vi "Ultrasonic.vi"(0 "COM":refnum<visa-resource-name>, 1 "Timeout (ms)":u32=500, 5 "Function":T2(ring)=enum."SendWaitRead", 7 "Send":string(combo), 9 "Baudrate":u32=115200, 11 "error in (no error)":errorcluster, 12 "Read regular":string="\n") -> (4 "ReceiveString":string, 6 "welding results  cluster":T1, 15 "error out":errorcluster)   [LabVIEW 2020, in "ultrasonic welding machine.lvlib"]
uses:
  ultrasonic welding machine.lvlib
  <vilib>/Instr/_visa.llb/VISA Set IO Buffer Mask.ctl
  <vilib>/Instr/_visa.llb/VISA Flush IO Buffer Mask.ctl
  <vilib>/Instr/_visa.llb/VISA Configure Serial Port (Instr).vi
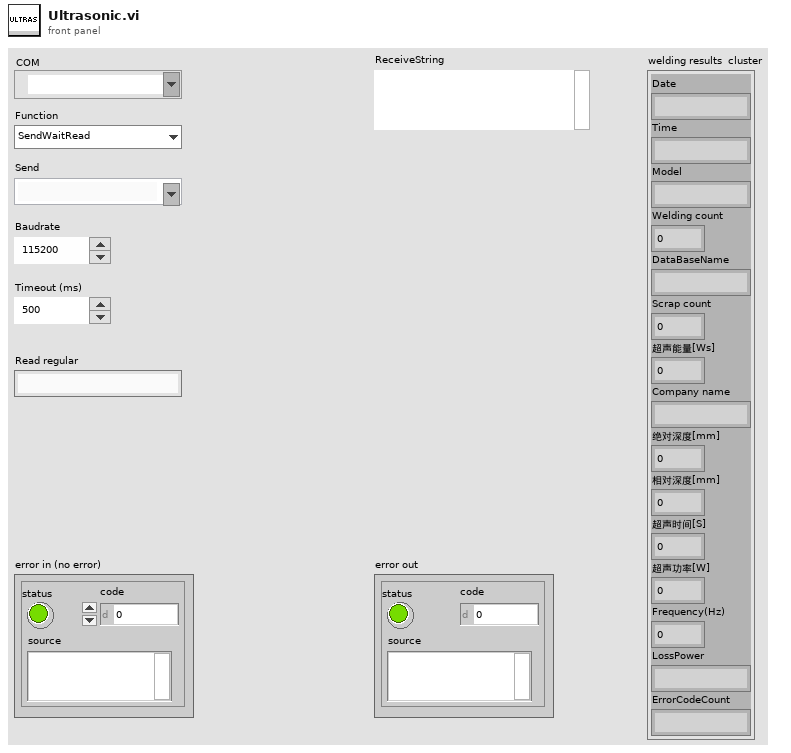
[diagram p1: front panel]
types:
  T1 = cluster{"Date":string, "Time":string, "Model":string, "Welding count ":i32, "DataBaseName":string, "Scrap count ":i32, "超声能量[Ws]":dbl, "Company name ":string, "绝对深度[mm]":dbl, "相对深度[mm]":dbl, "超声时间[S]":dbl, "超声功率[W]":dbl, "Frequency(Hz)":dbl, "LossPower":string, "ErrorCodeCount":string}
  T2 = enum16{"Open", "Close", "ClearBuffer", "Send", "Read", "SendWaitRead"}
  T3 = enum16{"Open", "Close", "ClearBuffer", "Send", "Read", "SendWaitRead", "SendCompare", "ReadCompare"}
  T4 = typedef "VISA Set IO Buffer Mask.ctl" = u16
  T5 = typedef "VISA Flush IO Buffer Mask.ctl" = u16
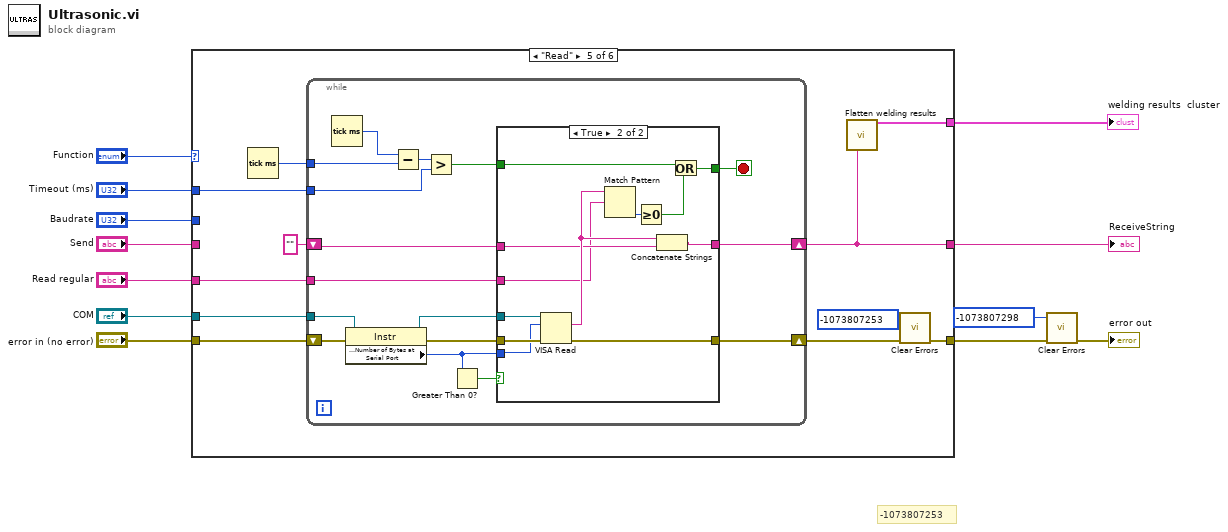
[diagram p0: block diagram]
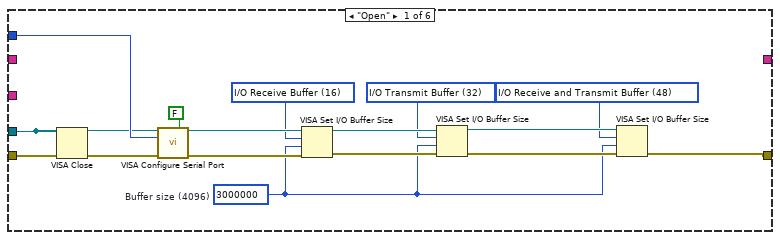
[diagram p2: hidden frame]
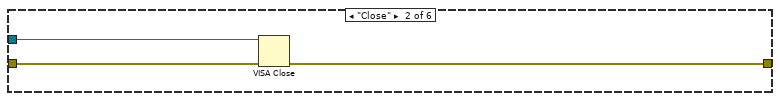
[diagram p3: hidden frame]
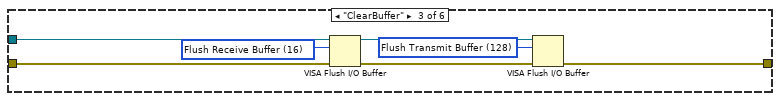
[diagram p4: hidden frame]
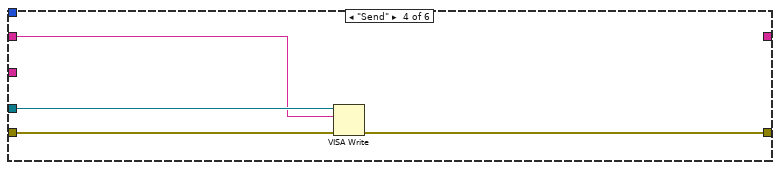
[diagram p5: hidden frame]
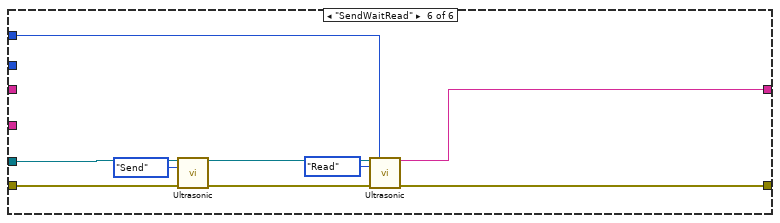
[diagram p7: hidden frame]
diagram:
  # "-1073807253"
  n1 = case shown="\"Read\"" "Function" {
    tunnel: "Send" -> [_ _ _ w39 _ _]
    tunnel: "error in (no error)" -> [w25 w30 w34 w41 w52 w88]
    tunnel: [w13 w29 w37 w42 w49 w91] -> w5
    tunnel: "COM" -> [w26 w31 w33 w40 w53 w89]
    tunnel: "Baudrate" -> [w28 _ _ _ _ _]
    tunnel: "Timeout (ms)" -> [_ _ _ _ w48 w84]
    tunnel: [_ _ _ _ w43 w87] -> w3
    tunnel: "Read regular" -> [_ _ _ _ w45 _]
    tunnel: [_ _ _ _ w44 _] -> w1
    frame "Open" {
      w14 = T4 16 items=["I/O Receive Buffer"=16, "I/O Transmit Buffer"=32, "I/O Receive and Transmit Buffer"=48] ("Mask")
      w15 = T4 48 items=["I/O Receive Buffer"=16, "I/O Transmit Buffer"=32, "I/O Receive and Transmit Buffer"=48] ("Mask")
      w16 = T4 32 items=["I/O Receive Buffer"=16, "I/O Transmit Buffer"=32, "I/O Receive and Transmit Buffer"=48] ("Mask")
      w17 = u32 3000000  # Buffer size (4096)
      n2 = VISA Close(VISA resource name=w26, error in (no error)=w25) -> (error out=w24:errorcluster)
      n3 = call-poly "VISA Configure Serial Port"("VISA resource name"=w26, "Enable Termination\nChar (T)"=FALSE ("Enable Termination\nChar (T)"), "baud rate (9600)"=w28, "error in (no error)"=w24) -> ("VISA resource name out"=w22:refnum<visa-resource-name>, "error out"=w23:errorcluster)  [unwired: 4 in, 6 out]
      n4 = VISA Set I/O Buffer Size(VISA resource name=w22, mask (16)=w14, size (4096)=w17, error in (no error)=w23) -> (VISA resource name out=w21:refnum<visa-resource-name>, error out=w19:errorcluster)
      n5 = VISA Set I/O Buffer Size(VISA resource name=w21, mask (16)=w16, size (4096)=w17, error in (no error)=w19) -> (VISA resource name out=w20:refnum<visa-resource-name>, error out=w18:errorcluster)
      n6 = VISA Set I/O Buffer Size(VISA resource name=w20, mask (16)=w15, size (4096)=w17, error in (no error)=w18) -> (error out=w13:errorcluster)  [unwired: 1 out]
    }
    frame "Close" {
      n7 = VISA Close(VISA resource name=w31, error in (no error)=w30) -> (error out=w29:errorcluster)
    }
    frame "ClearBuffer" {
      w36 = T5 16 items=["Flush Receive Buffer"=16, "Write Transmit Buffer to Device"=32, "Flush Receive Buffer (No I/O)"=64, "Flush Transmit Buffer"=128] ("Mask")
      w38 = T5 128 items=["Flush Receive Buffer"=16, "Write Transmit Buffer to Device"=32, "Flush Receive Buffer (No I/O)"=64, "Flush Transmit Buffer"=128] ("Mask")
      n8 = VISA Flush I/O Buffer(VISA resource name=w33, mask (16)=w36, error in (no error)=w34) -> (VISA resource name out=w32:refnum<visa-resource-name>, error out=w35:errorcluster)
      n9 = VISA Flush I/O Buffer(VISA resource name=w32, mask (16)=w38, error in (no error)=w35) -> (error out=w37:errorcluster)  [unwired: 1 out]
    }
    frame "Send" {
      n10 = VISA Write(VISA resource name=w40, write buffer=w39, error in (no error)=w41) -> (error out=w42:errorcluster)  [unwired: 2 out]
    }
    frame "Read" {
      n11 = Tick Count (ms)() -> (millisecond timer value=w47:u32)
      n12 = while {
        tunnel: w53 -> [w69]
        shift-right: [w64] -> w50
        shift-left: w52 -> [w56]
        tunnel: w48 -> [w59]
        tunnel: w47 -> [w61]
        shift-right: [w65] -> w43
        shift-left: "" ("read buffer") -> [w57]
        tunnel: w45 -> [w54]
        stop <- w63 stop-if-true
        n13 = Tick Count (ms)() -> (millisecond timer value=w62:u32)
        n14 = property class="Instr"(reference=w69, error in=w56) -> (reference out=w68:refnum<visa-resource-name>, error out=w55:errorcluster, "Serial Settings:Number of Bytes at Serial Port"=w67:u32)
        n15 = Subtract(x=w62, y=w61) -> (x-y=w60:u32)
        n16 = Greater?(x=w60, y=w59) -> (0:w58:bool)
        n17 = Greater Than 0?(x=w67) -> (x > 0?=w66:bool)
        n18 = case shown="True" w66 {
          tunnel: [w71 w83] -> w64
          tunnel: w55 -> [w71 w82]
          tunnel: w68 -> [_ w81]
          tunnel: [_ w75] -> w65
          tunnel: w67 -> [_ w73]
          tunnel: [w70 w78] -> w63
          tunnel: w58 -> [w70 w76]
          tunnel: w57 -> [_ w74]
          tunnel: w54 -> [_ w72]
          frame False {
          }
          frame True {
            n19 = VISA Read(VISA resource name=w81, byte count=w73, error in (no error)=w82) -> (read buffer=w80:string, error out=w83:errorcluster)  [unwired: 2 out]
            n20 = Match Pattern(string=w80, regular expression=w72) -> (offset past match=w79:i32)  [unwired: 1 in, 3 out]
            n21 = Greater Or Equal To 0?(x=w79) -> (x >= 0?=w77:bool)
            n22 = Concatenate Strings(w80, w74) -> (w75:string)
            n23 = Or(x=w76, y=w77) -> (x .or. y?=w78:bool)
          }
        }
      }
      n24 = call "Flatten welding results.vi"("welding results"=w43) -> ("welding results  cluster"=w44:T1)  [unwired: 14 in]
      n25 = call <vilib>:"Clear Errors.vi"("error in (no error)"=w50, "specific error code to clear (0: all)"=-1073807253) -> ("error out"=w49:errorcluster)  [unwired: 4 in, 1 out]
    }
    frame "SendWaitRead" {
      n26 = call "Ultrasonic.vi"("COM"=w89, "Function"=T3."Send", "error in (no error)"=w88) -> ("error out"=w90:errorcluster)  [unwired: 10 in, 2 out]
      n27 = call "Ultrasonic.vi"("COM"=w89, "Timeout (ms)"=w84, "Function"=T3."Read", "error in (no error)"=w90) -> ("ReceiveString"=w87:string, "error out"=w91:errorcluster)  [unwired: 9 in, 1 out]
    }
  }
  "ReceiveString" <- w3
  "welding results  cluster" <- w1
  n28 = call <vilib>:"Clear Errors.vi"("error in (no error)"=w5, "specific error code to clear (0: all)"=-1073807298) -> ("error out"=→"error out":errorcluster)  [unwired: 4 in, 1 out]
